vi "get Non Solid.vi"(11 "Element in":refnum<class "Element.lvclass">) -> (3 "Non Solid":bool)   [LabVIEW 2021, in "Element.lvclass"]
uses:
  Element.lvclass
  Element.lvclass/Element.ctl
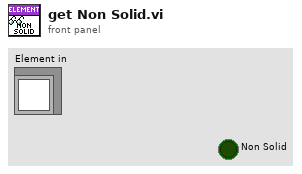
[diagram p1: front panel]
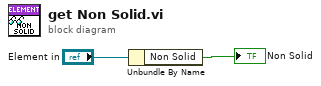
[diagram p0: block diagram]
diagram:
  n1 = Unbundle By Name("Element in") -> ("Non Solid"=→"Non Solid":bool)
